vi "DecimalToBCD.vi"(11 "U8":u8 format="%02d") -> (3 "BCD":u8 format="%0d")   [LabVIEW 2020]
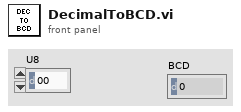
[diagram p1: front panel]
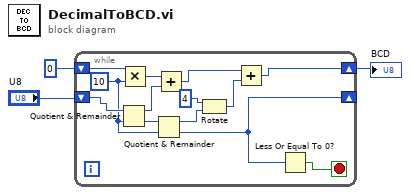
[diagram p0: block diagram]
diagram:
  n1 = while {
    shift-right: [w9] -> _
    shift-left: "U8" -> [w14]
    shift-right: [w4] -> w1
    shift-left: u8 0 ("lower limit") -> [w15]
    stop <- w16 stop-if-true
    w10 = u8 10 ("y")
    n2 = Quotient & Remainder(x=w14, y=w10) -> (x-y*floor(x/y)=w12:u8, floor(x/y)=w11:u8)
    n3 = Multiply(x=w15, y=w10) -> (x*y=w13:u8)
    n4 = Quotient & Remainder(x=w11, y=w10) -> (x-y*floor(x/y)=w7:u8, floor(x/y)=w9:u8)
    n5 = Add(x=w13, y=w12) -> (x+y=w6:u8)
    n6 = Rotate(1:w7, 2:u8 4 ("x")) -> (0:w5:u8)
    n7 = Add(x=w6, y=w5) -> (x+y=w4:u8)
    n8 = Less Or Equal To 0?(x=w9) -> (x <= 0?=w16:bool)
  }
  "BCD" <- w1
